vi "Rohde & Schwarz VNA Set Frequency On-Off.vi"(7 "Rohde & Schwarz VNA":T1, 8 "error in (no error)":errorcluster, 10 "Blank Frequencies (F)":bool, 11 "VISA Resource Name":refnum<visa-resource-name>) -> (0 "error out":errorcluster, 3 "dup VISA Resource Name":refnum<visa-resource-name>)   [LabVIEW 2011]
doc: "This VI for the HP8753B Network Analyzers reads the stimulus values. Except when performing log sweeps and freq list sweeps, this VI uses the start and stop values and the number of points to calcuate the stimulus values."
uses:
  TypeDefs/Rohde & Schwarz VNA Instrument Info.ctl
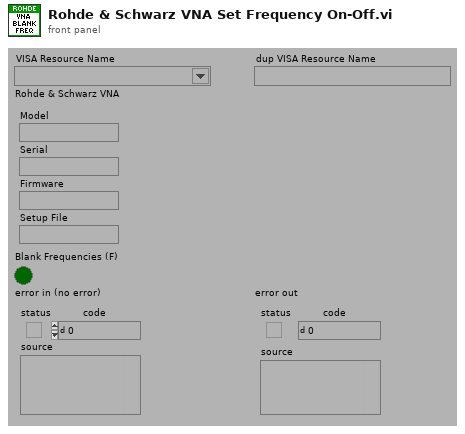
[diagram p1: front panel]
types:
  T1 = typedef "Rohde & Schwarz VNA Instrument Info.ctl" = cluster{"Model":string, "Serial":string, "Firmware":string, "Setup File":string}
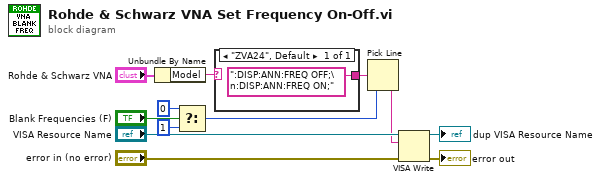
[diagram p0: block diagram]
diagram:
  n1 = Unbundle By Name("Rohde & Schwarz VNA") -> ("Model"=w7:string)
  n2 = Select(t=0, s="Blank Frequencies (F)", f=1) -> (s? t:f=w3:i32)
  n3 = case shown="\"ZVA24\", Default" w7 {
    tunnel: [":DISP:ANN:FREQ OFF;\n:DISP:ANN:FREQ ON;"] -> w2
    frame "ZVA24", Default {
    }
  }
  n4 = Pick Line(multi-line string=w2, line index=w3) -> (output string=w1:string)  [unwired: 1 out]
  n5 = VISA Write(VISA resource name="VISA Resource Name", write buffer=w1, error in (no error)="error in (no error)") -> (VISA resource name out=→"dup VISA Resource Name":refnum<visa-resource-name>, error out=→"error out":errorcluster)  [unwired: 1 out]
